vi "Globals (private).vi"() -> ()   [LabVIEW 2015, in "SB SubVIs.lvlib"]
uses:
  SB SubVIs.lvlib
  Square/Square.lvclass
panel:
  in  "Round":i32
  in  "Winning":i32
  in  "Board Size":i32
  in  "Time Limit":i32
  in  "Start Time":timestamp
  out "Players":T1(array[cluster])
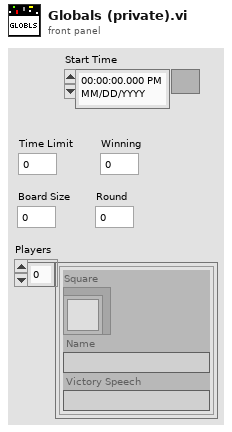
[diagram p1: front panel]
types:
  T1 = cluster{"Square":refnum<class "Square.lvclass">, "Name":string, "Victory Speech":string}[]
diagram:
